vi "Column size.vi"() -> ()   [LabVIEW 2022 SP3]
panel:
  out "Column size":i32
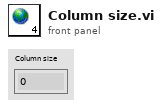
[diagram p1: front panel]
diagram:
